vi "Game.vi"() -> ()   [LabVIEW 2025]
uses:
  Controls/Game.ctl
  Controls/Player.ctl
  <vilib>/Utility/miscctls.llb/LVPositionTypeDef.ctl
  38faf71d-537f-4ad3-ba2d-5a527e0ddfb2.vi
panel:
  out "CurrentPlayer":i32
  out "Hand3":u16[](array[ring]) caption="Tiles"
  out "River4":u16[][](array[ring]) caption="Tiles"
  out "Door4":u16[](array[ring]) caption="Tiles"
  out "Hand4":u16[](array[ring]) caption="Tiles"
  out "Door3":u16[](array[ring]) caption="Tiles"
  out "River 3":u16[][](array[ring]) caption="Tiles"
  in  "Chi 3":bool
  in  "Chi 2":bool
  in  "Chi 1":bool
  in  "Cancel":bool
  in  "Hu":bool
  in  "Kung":bool
  in  "Pong":bool
  in  "Chi":bool
  out "Players":T1[](array[typedef])
  out "Game":T2
  out "River1":u16[][](array[ring]) caption="Tiles"
  in  "Buttons":bool[](array[boolean])=[FALSE, FALSE, FALSE, FALSE, FALSE, FALSE, FALSE, FALSE, FALSE, FALSE, FALSE, FALSE, FALSE, FALSE, FALSE, FALSE, FALSE]
  out "Hand1":u16[](array[ring])
  out "River2":u16[][](array[ring]) caption="Tiles"
  out "Door2":u16[](array[ring]) caption="Tiles"
  out "Hand2":u16[](array[ring]) caption="Tiles"
  out "Door1":u16[](array[ring]) caption="Tiles"
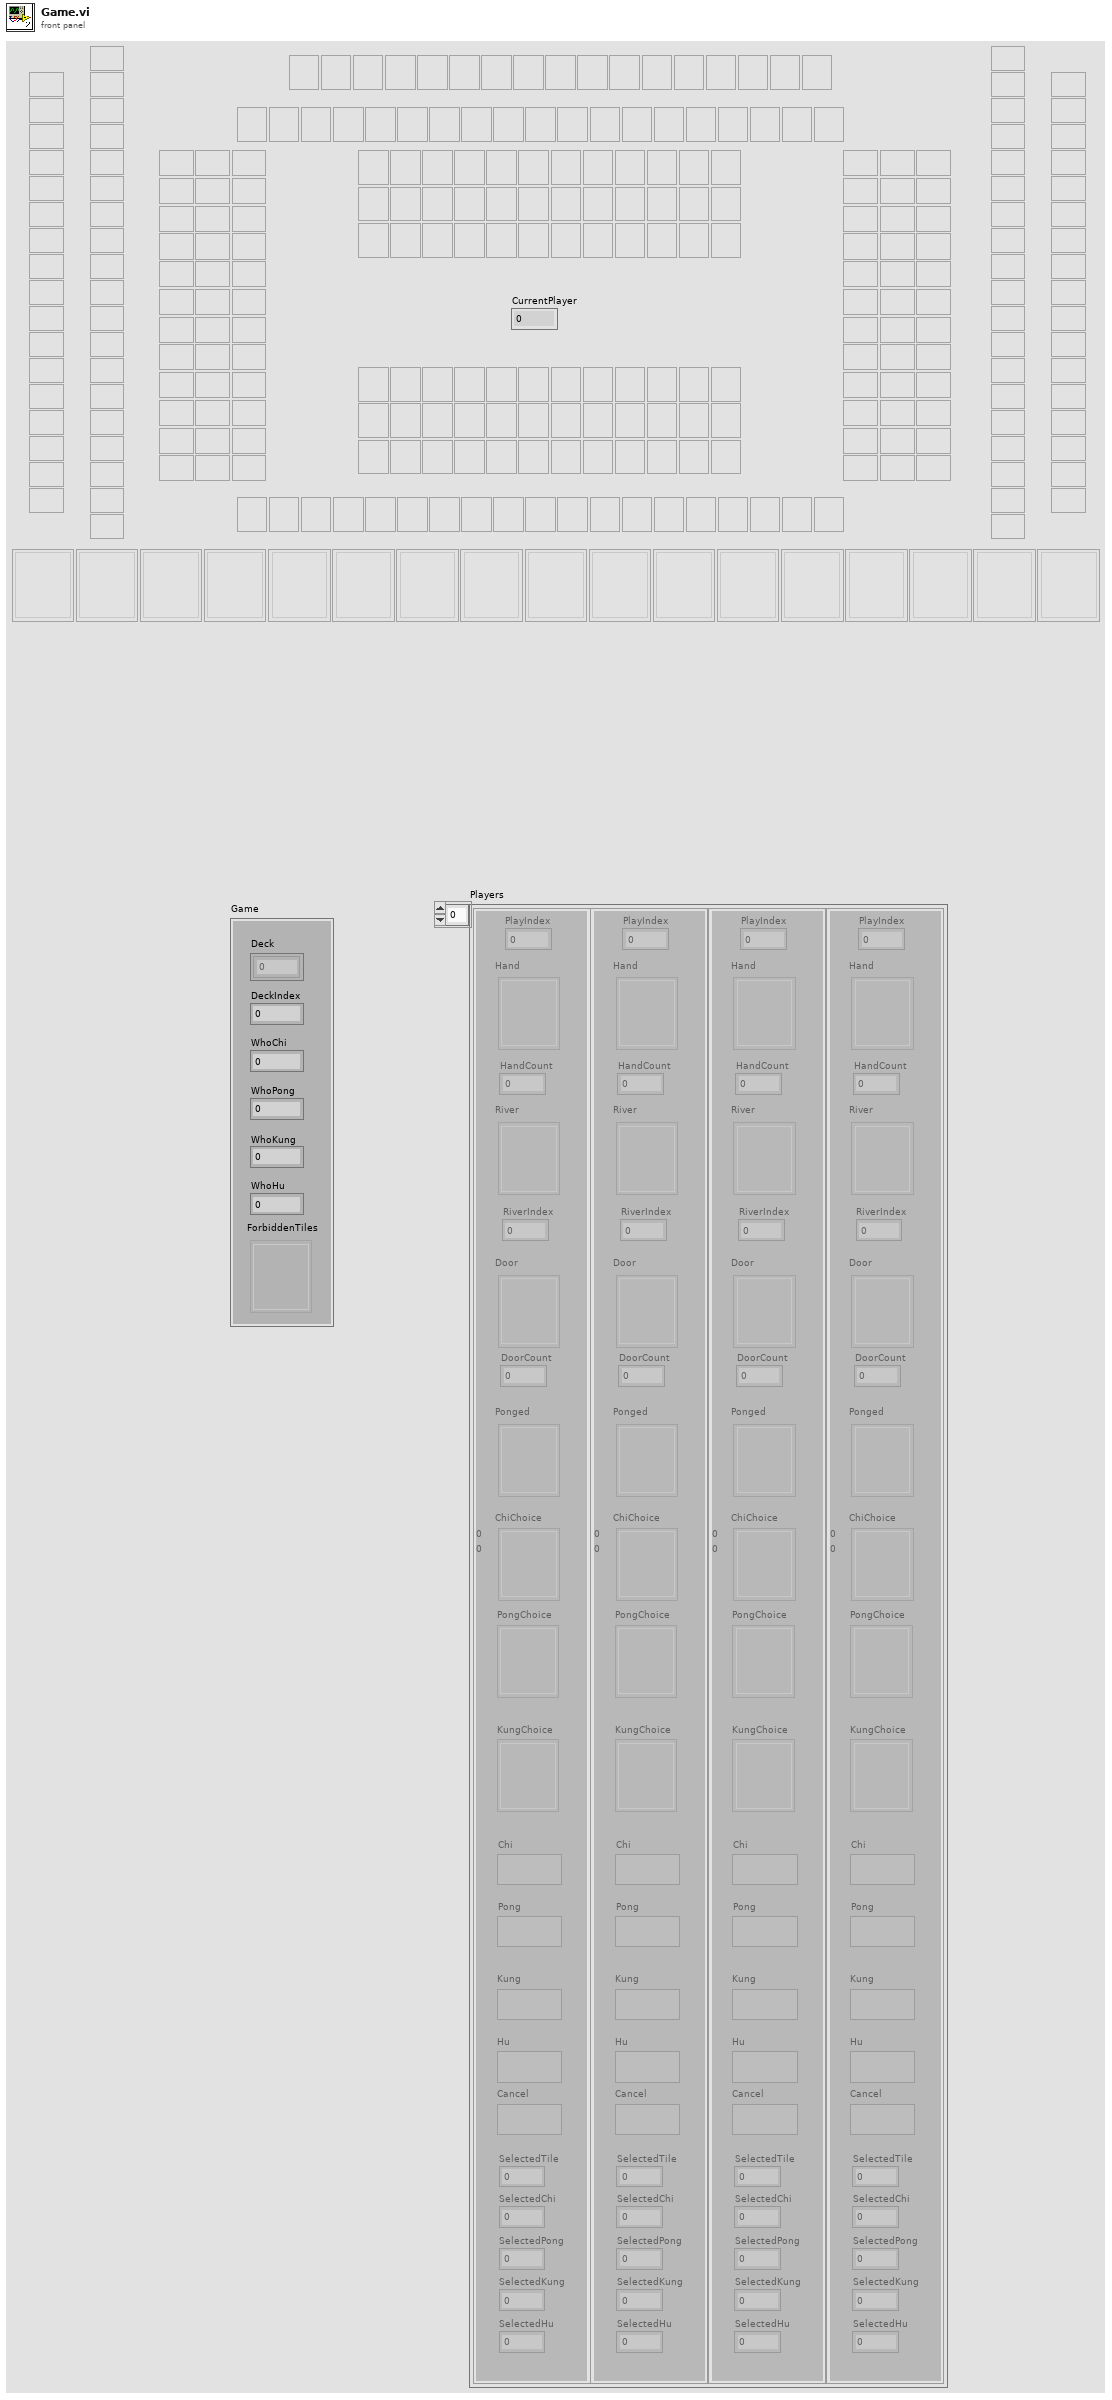
[diagram p1: front panel]
types:
  T1 = typedef "Player.ctl" = cluster{"PlayIndex":u16, "Hand":u16[], "HandCount":u16, "RiverIndex":u16, "Door":u16[], "DoorCount":u16, "Ponged":u16[], "ChiChoice":u16[][], "River":u16[][], "Chi":bool, "Pong":bool, "Kung":bool, "Hu":bool, "Cancel":bool, "PongChoice":u16, "KungChoice":u16, "SelectedTile":i16, "SelectedChi":i16, "SelectedPong":i16, "SelectedKung":i16, "SelectedHu":i16}
  T2 = typedef "Game.ctl" = cluster{"DeckIndex":u16, "Deck":u16[], "WhoChi":u16, "WhoPong":u16, "WhoKung":u16, "WhoHu":u16, "ForbiddenTiles":u16[]}
  T3 = enum16{"Game Start", "DeckSetup", "PlayerSetup", "Deal", "Game End", "Draw", "Wait", "WaitKung", "Throw", "Chi", "Pong", "Kung", "Hu", "Interrupt0", "Interrupt1", "Interrupt2", "Interrupt3", "Chi?", "Pong?", "Kung?", "Hu?"}
  T4 = enum8{"Enabled", "Disabled", "Disabled and Grayed Out"}
  T5 = typedef "LVPositionTypeDef.ctl" = cluster{"Left":i32, "Top":i32}
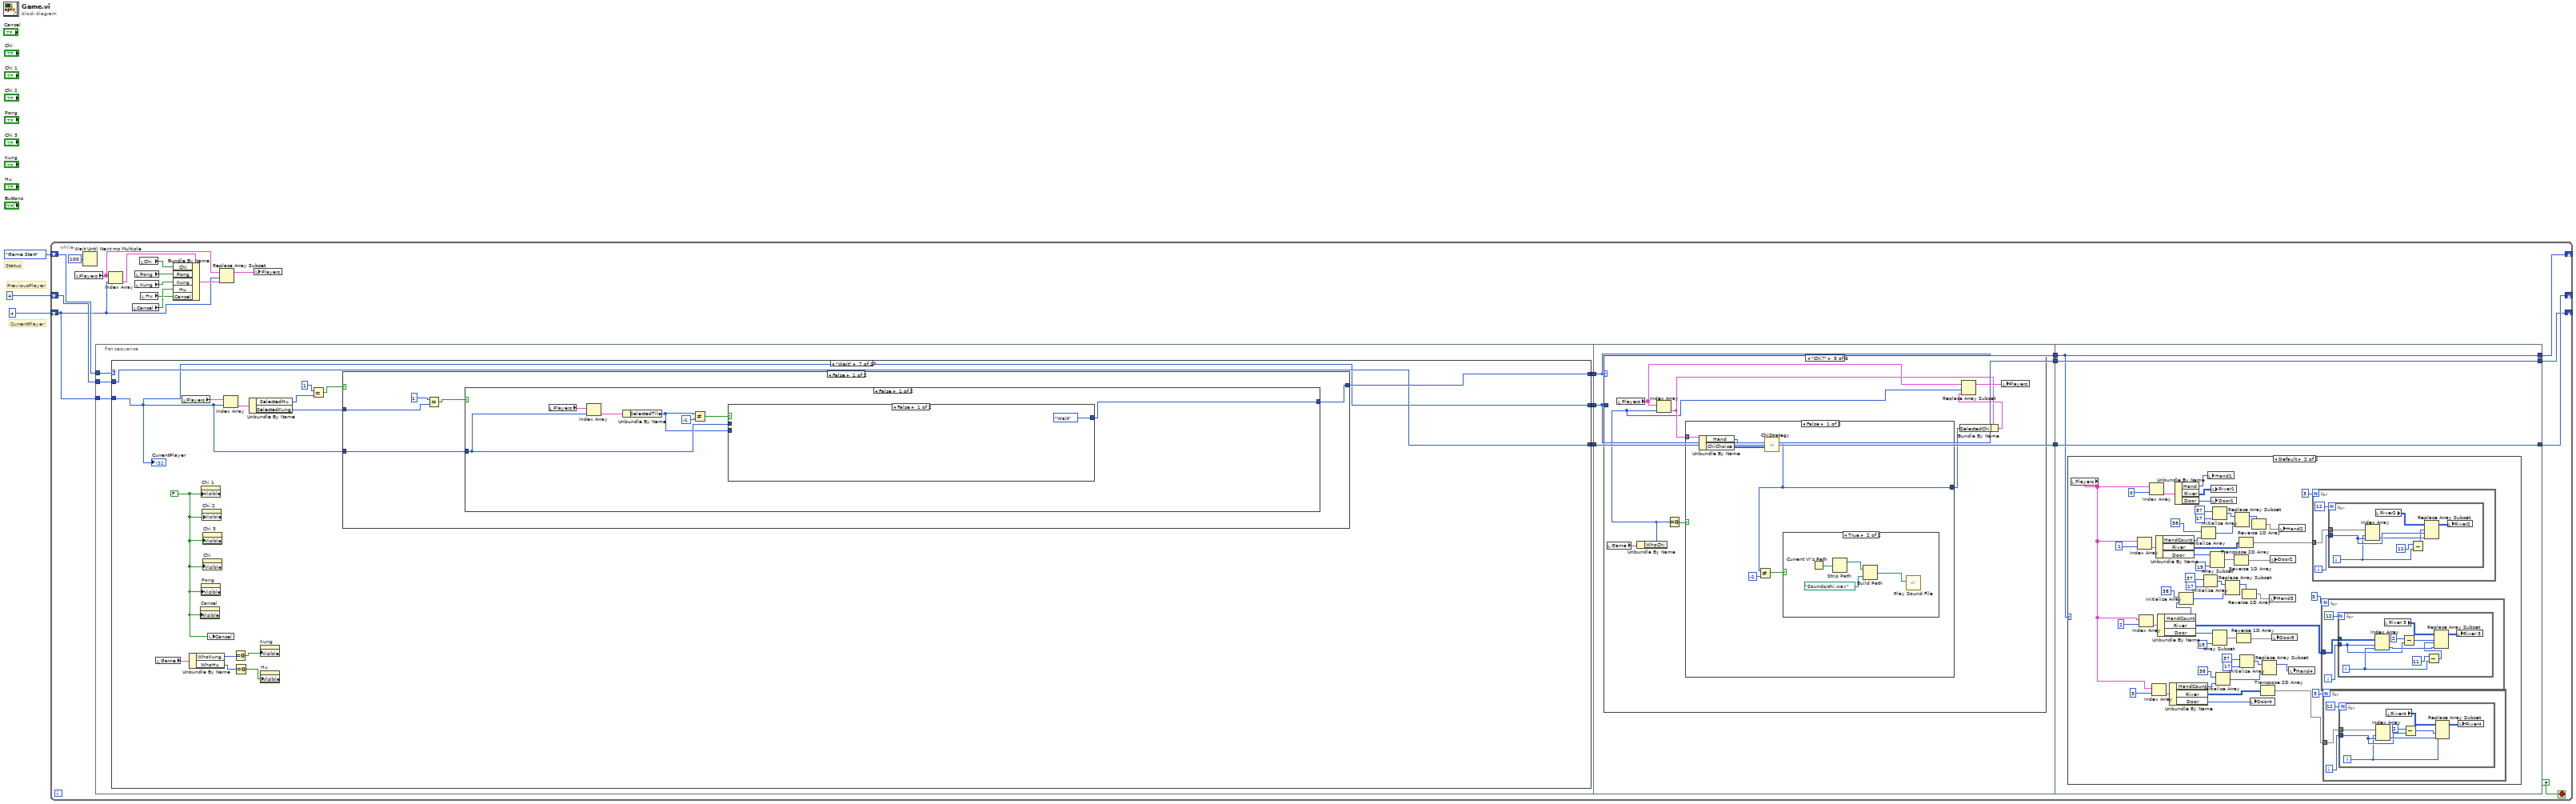
[diagram p0: block diagram]
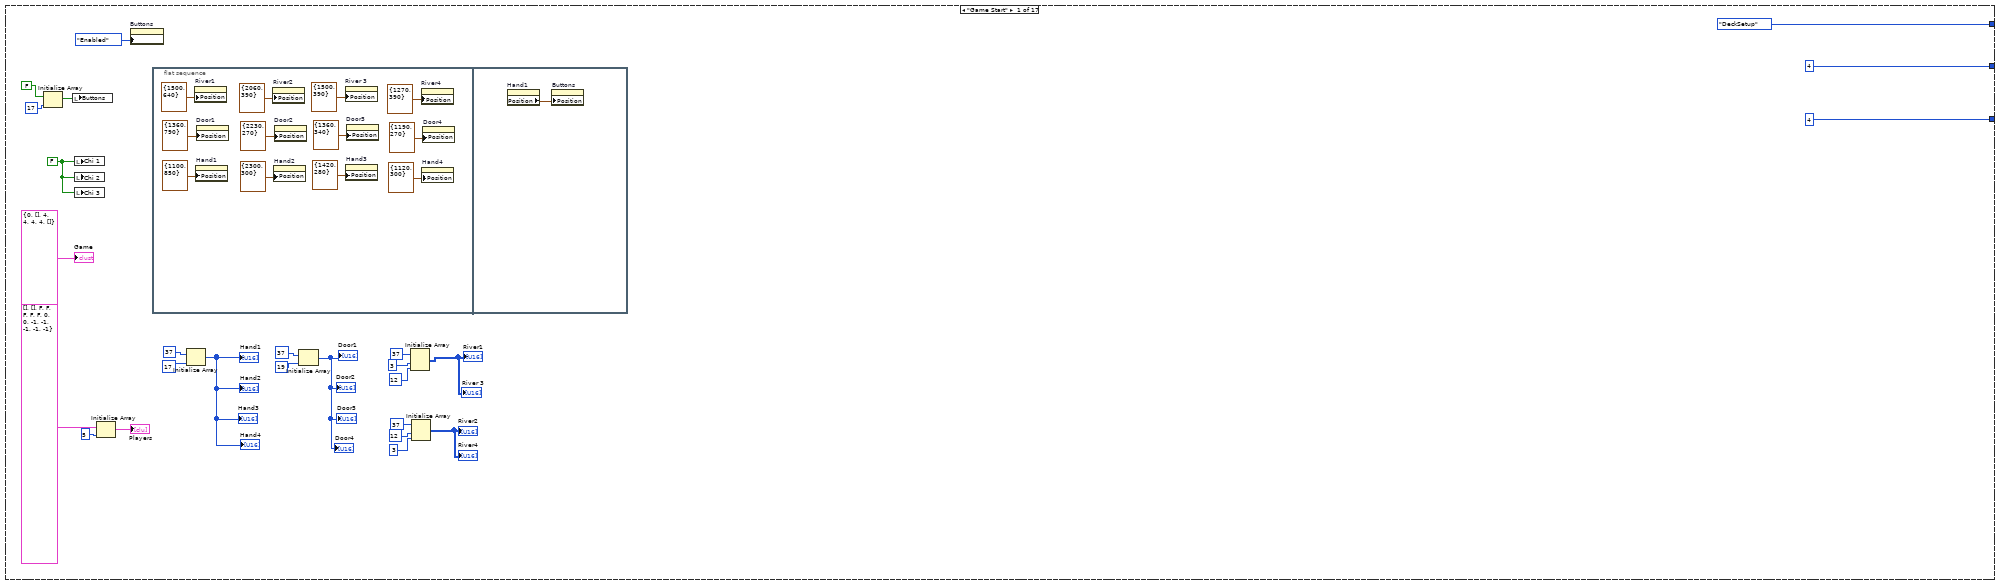
[diagram p2: hidden frame]
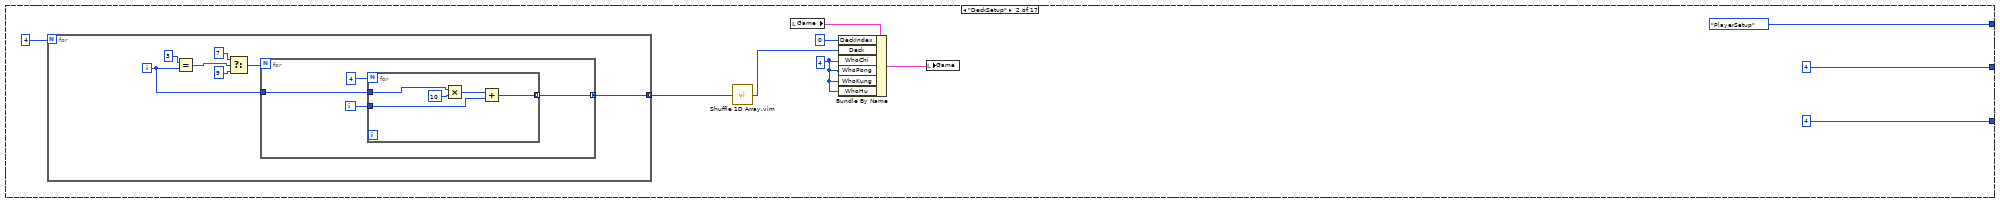
[diagram p3: hidden frame]
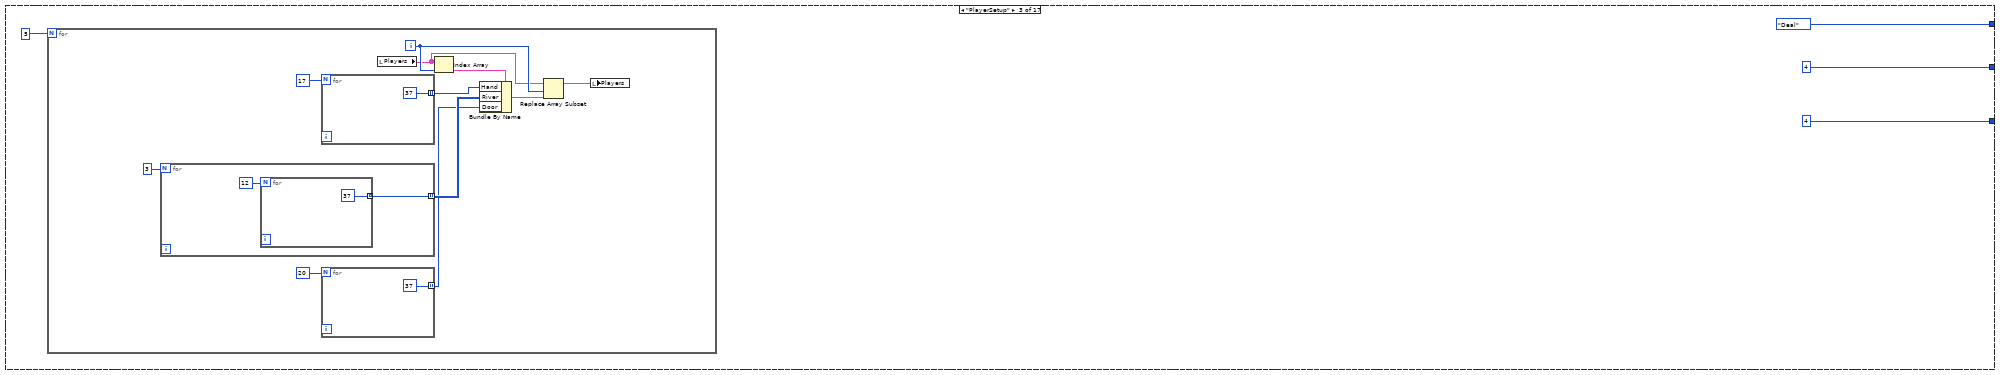
[diagram p4: hidden frame]
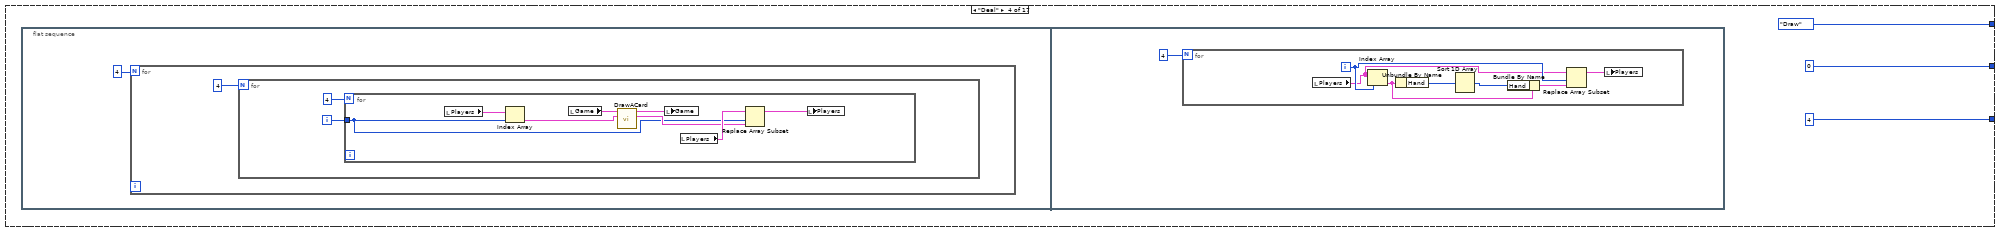
[diagram p5: hidden frame]
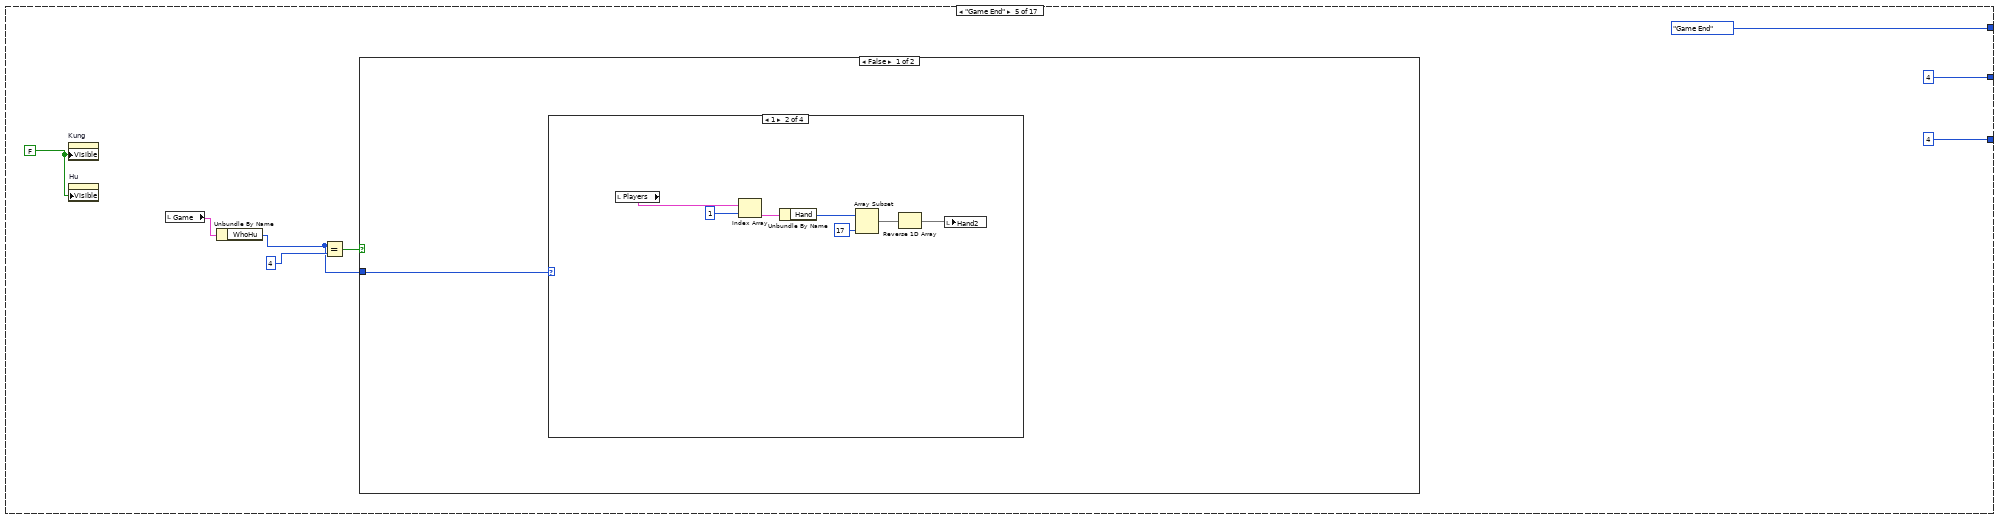
[diagram p6: hidden frame]
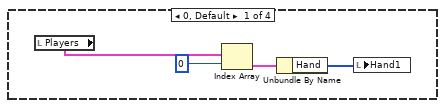
[diagram p7: hidden frame]
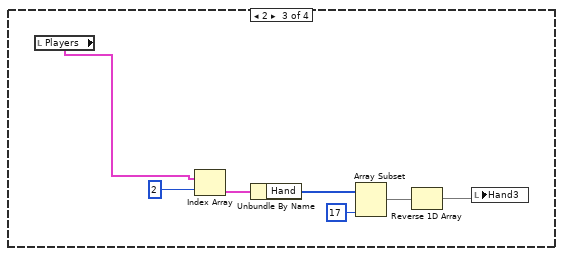
[diagram p8: hidden frame]
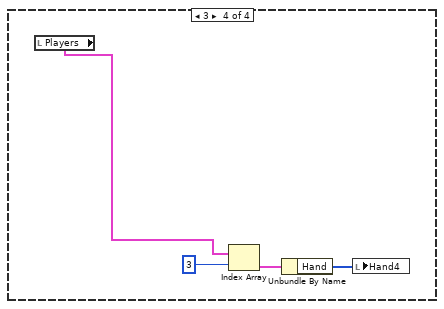
[diagram p9: hidden frame]
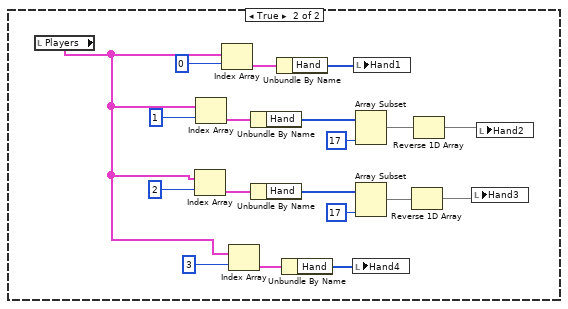
[diagram p10: hidden frame]
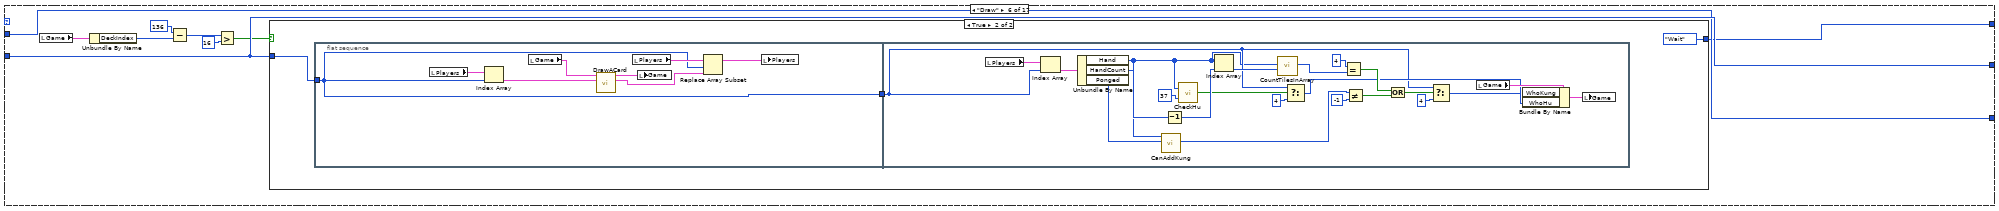
[diagram p11: hidden frame]
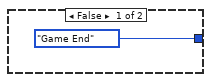
[diagram p12: hidden frame]
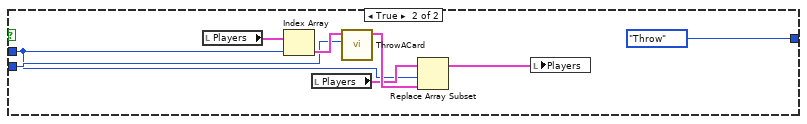
[diagram p13: hidden frame]
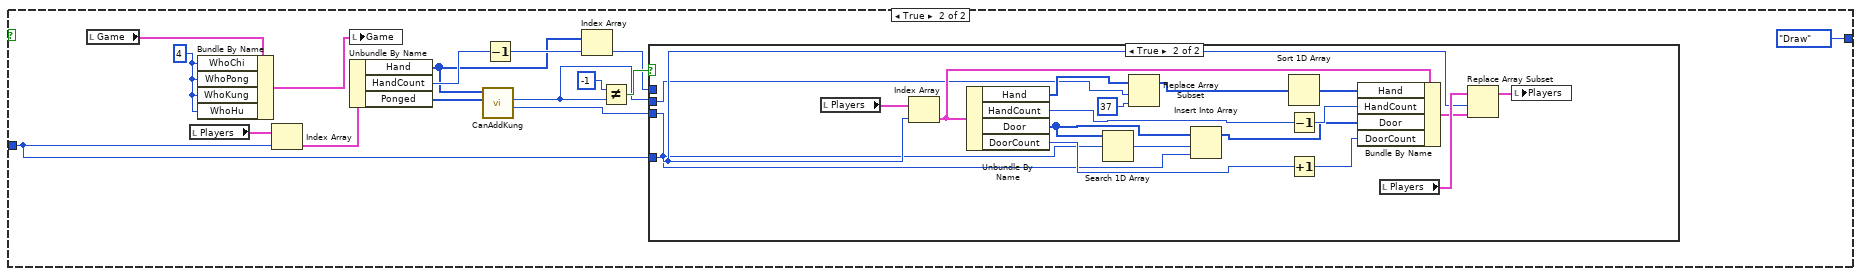
[diagram p14: hidden frame]
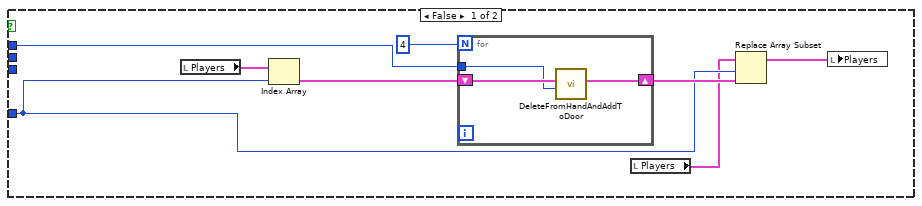
[diagram p15: hidden frame]
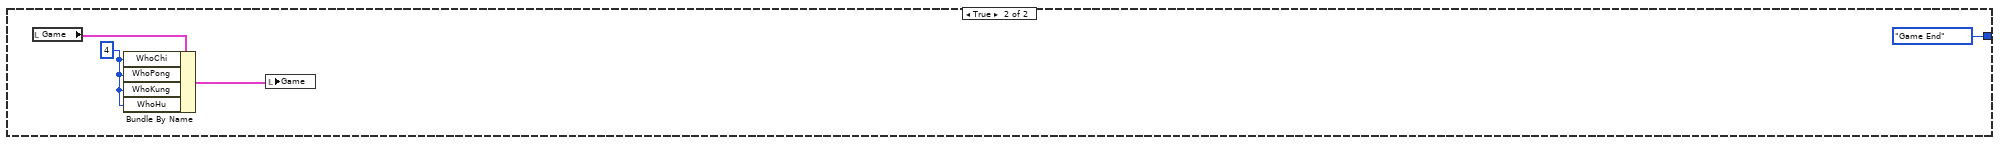
[diagram p16: hidden frame]
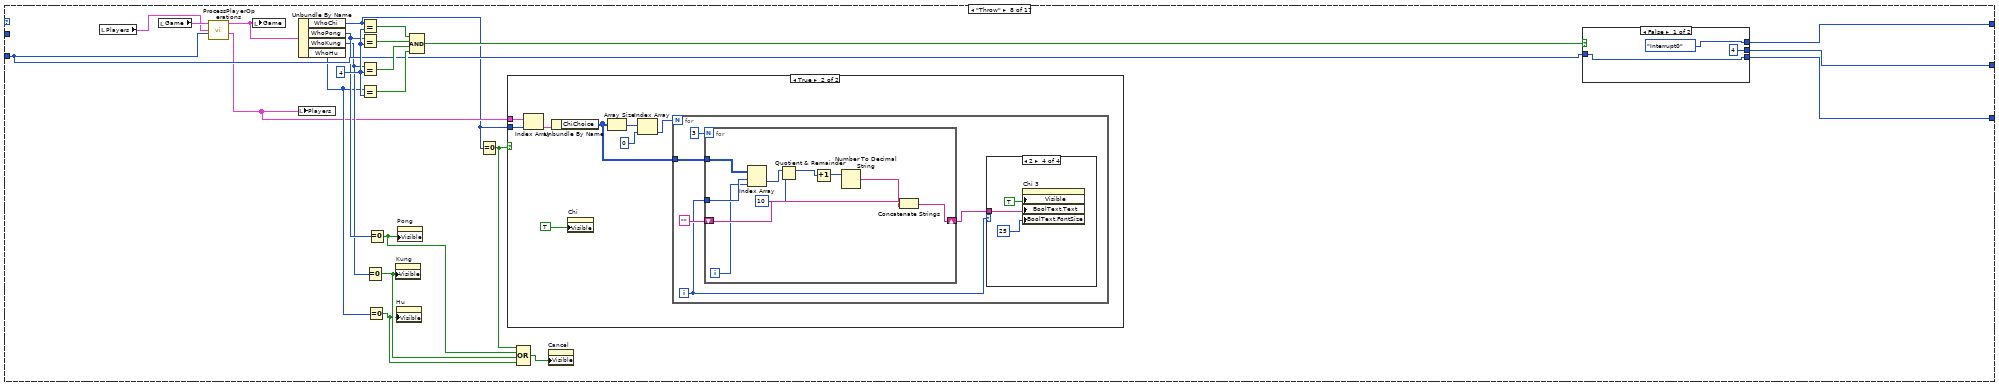
[diagram p17: hidden frame]
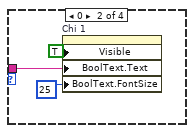
[diagram p20: hidden frame]
diagram:
  # "PreviousPlayer"
  # "CurrentPlayer"
  # "Status"
  n1 = while {
    shift-right: [w21] -> _
    shift-left: T3."Game Start" -> [w11]
    shift-right: [w22] -> _
    shift-left: 4 -> [w10]
    shift-right: [w23] -> _
    shift-left: 4 -> [w24]
    stop <- FALSE stop-if-true
    n2 = local read "Players"() -> (w18:T1[])
    n3 = Wait Until Next ms Multiple(millisecond multiple=100) -> ()  [unwired: 1 out]
    n4 = flat-sequence {
      tunnel: w24 -> [w32]
      tunnel: w11 -> [w29]
      tunnel: w10 -> [w28]
      tunnel: [w31] -> w9
      tunnel: [w27] -> w8
      tunnel: [w30] -> w7
      tunnel: w9 -> [w573]
      tunnel: w8 -> [w572]
      tunnel: w7 -> [w574]
      tunnel: [w573] -> w6
      tunnel: [w572] -> w5
      tunnel: [w574] -> w4
      tunnel: [w779] -> w21
      tunnel: [w780] -> w22
      tunnel: [w781] -> w23
      tunnel: w6 -> [w781]
      tunnel: w5 -> [w780]
      tunnel: w4 -> [w779]
      frame #0 {
        n5 = case shown="\"Wait\"" w29 {
          tunnel: [T3."DeckSetup" T3."PlayerSetup" T3."Deal" T3."Draw" T3."Game End" w191 w249 w336 w385 w396 w407 w419 w433 w484 w522 w556 T3."Game End"] -> w30
          tunnel: w28 -> [_ _ _ _ _ w199 w246 w334 _ _ _ _ w431 w480 w518 w552 _]
          tunnel: w32 -> [_ _ _ _ _ w198 w248 _ w386 w395 w409 w418 w434 w481 w519 w553 _]
          tunnel: [4 4 4 4 4 w198 w248 w335 w386 w395 w409 w420 w432 w483 w521 w555 4] -> w31
          tunnel: [4 4 4 0 4 w199 w246 w337 w384 w397 w406 w417 w436 w482 w520 w554 4] -> w27
          frame "Game Start" {
            w51 = FALSE
            n6 = Initialize Array(FALSE, 17) -> (w48:bool[])
            n7 = local write "Buttons"(w48) -> ()
            n8 = local write "Chi 1"(w51) -> ()
            n9 = local write "Chi 2"(w51) -> ()
            n10 = local write "Chi 3"(w51) -> ()
            n11 = Initialize Array(T1 {"PlayIndex"=0, "Hand"=[], "HandCount"=0, "RiverIndex"=0, "Door"=[], "DoorCount"=0, "Ponged"=[], "ChiChoice"=[], "River"=[], "Chi"=FALSE, "Pong"=FALSE, "Kung"=FALSE, "Hu"=FALSE, "Cancel"=FALSE, "PongChoice"=0, "KungChoice"=0, "SelectedTile"=-1, "SelectedChi"=-1, "SelectedPong"=-1, "SelectedKung"=-1, "SelectedHu"=-1} ("element"), 5) -> (→"Players":T1[])
            n12 = property on="Buttons" class="Arr (strict)"("DisabledEnum"=T4."Enabled" ("Disabled")) -> ()  [unwired: 2 in, 2 out]
            n13 = flat-sequence {
              frame #0 {
                n14 = property on="River1" class="Arr (strict)"("Position"=T5 {"Left"=1500, "Top"=640}) -> ()  [unwired: 2 in, 2 out]
                n15 = property on="Hand1" class="Arr (strict)"("Position"=T5 {"Left"=1100, "Top"=850}) -> ()  [unwired: 2 in, 2 out]
                n16 = property on="Door1" class="Arr (strict)"("Position"=T5 {"Left"=1360, "Top"=790}) -> ()  [unwired: 2 in, 2 out]
                n17 = property on="River2" class="Arr (strict)"("Position"=T5 {"Left"=2060, "Top"=390}) -> ()  [unwired: 2 in, 2 out]
                n18 = property on="Hand2" class="Arr (strict)"("Position"=T5 {"Left"=2300, "Top"=300}) -> ()  [unwired: 2 in, 2 out]
                n19 = property on="Door2" class="Arr (strict)"("Position"=T5 {"Left"=2230, "Top"=270}) -> ()  [unwired: 2 in, 2 out]
                n20 = property on="River 3" class="Arr (strict)"("Position"=T5 {"Left"=1500, "Top"=390}) -> ()  [unwired: 2 in, 2 out]
                n21 = property on="Hand3" class="Arr (strict)"("Position"=T5 {"Left"=1420, "Top"=280}) -> ()  [unwired: 2 in, 2 out]
                n22 = property on="Door3" class="Arr (strict)"("Position"=T5 {"Left"=1360, "Top"=340}) -> ()  [unwired: 2 in, 2 out]
                n23 = property on="River4" class="Arr (strict)"("Position"=T5 {"Left"=1270, "Top"=390}) -> ()  [unwired: 2 in, 2 out]
                n24 = property on="Hand4" class="Arr (strict)"("Position"=T5 {"Left"=1120, "Top"=300}) -> ()  [unwired: 2 in, 2 out]
                n25 = property on="Door4" class="Arr (strict)"("Position"=T5 {"Left"=1190, "Top"=270}) -> ()  [unwired: 2 in, 2 out]
              }
              frame #1 {
                n26 = property on="Hand1" class="Arr (strict)"() -> ("Position"=w71:T5)  [unwired: 2 in, 2 out]
                n27 = property on="Buttons" class="Arr (strict)"("Position"=w71) -> ()  [unwired: 2 in, 2 out]
              }
            }
            n28 = Initialize Array(37, 17) -> (→"Hand1" →"Hand3" →"Hand4" →"Hand2":i32[])
            n29 = Initialize Array(37, 19) -> (→"Door3" →"Door1" →"Door4" →"Door2":i32[])
            n30 = Initialize Array(37, 3, 12) -> (→"River1" →"River 3":i32[][])
            n31 = Initialize Array(37, 12, 3) -> (→"River2" →"River4":i32[][])
            "Game" <- T2 {"DeckIndex"=0, "Deck"=[], "WhoChi"=4, "WhoPong"=4, "WhoKung"=4, "WhoHu"=4, "ForbiddenTiles"=[]} ("Game")
          }
          frame "DeckSetup" {
            w72 = 4
            n32 = for {
              N: 4 -> [_]
              tunnel: [w85] -> w81 mode=concatenating
              i -> [w83]
              n33 = Equal?(x=3, y=w83) -> (x = y?=w84:bool)
              n34 = Select(t=7, s=w84, f=9) -> (s? t:f=w87:i32)
              n35 = for {
                N: w87 -> [_]
                tunnel: w83 -> [w92]
                tunnel: [w90] -> w85 mode=concatenating
                i -> [w91]
                n36 = for {
                  N: 4 -> [_]
                  tunnel: w92 -> [w95]
                  tunnel: w91 -> [w94]
                  tunnel: [w93] -> w90 mode=indexing
                  n37 = Multiply(x=w95, y=10) -> (x*y=w97:i32)
                  n38 = Add(x=w97, y=w94) -> (x+y=w93:i32)
                }
              }
            }
            n39 = call "Shuffle 1D Array.vim"("array"=w81) -> ("shuffled array"=w78:i32[])  [unwired: 4 in]
            n40 = local read "Game"() -> (w79:T2)
            n41 = Bundle By Name(cluster=w79, "DeckIndex"=0, "Deck"=w78, "WhoChi"=w72, "WhoPong"=w72, "WhoKung"=w72, "WhoHu"=w72) -> (w80:T2)
            n42 = local write "Game"(w80) -> ()
          }
          frame "PlayerSetup" {
            n43 = for {
              N: 5 -> [_]
              i -> [w109]
              n44 = for {
                N: 3 -> [_]
                tunnel: [w115] -> w105 mode=indexing
                n45 = for {
                  N: 12 -> [_]
                  tunnel: [37] -> w115 mode=indexing
                }
              }
              n46 = for {
                N: 17 -> [_]
                tunnel: [37] -> w106 mode=indexing
              }
              n47 = for {
                N: 20 -> [_]
                tunnel: [37] -> w102 mode=indexing
              }
              n48 = local read "Players"() -> (w108:T1[])
              n49 = Index Array(array=w108, index=w109) -> (element=w112:T1)
              n50 = Bundle By Name(cluster=w112, "Hand"=w106, "River"=w105, "Door"=w102) -> (w111:T1)
              n51 = Replace Array Subset(array=w108, new element=w111, index=w109) -> (w110:T1[])
              n52 = local write "Players"(w110) -> ()
            }
          }
          frame "Deal" {
            n53 = flat-sequence {
              frame #0 {
                n54 = for {
                  N: 4 -> [_]
                  n55 = for {
                    N: 4 -> [_]
                    i -> [w123]
                    n56 = for {
                      N: 4 -> [_]
                      tunnel: w123 -> [w127]
                      n57 = local read "Players"() -> (w126:T1[])
                      n58 = Index Array(array=w126, index=w127) -> (element=w125:T1)
                      n59 = local read "Game"() -> (w128:T2)
                      n60 = call "DrawACard.vi"("Player"=w125, "Game"=w128) -> ("NewPlayer"=w130:T1, "NewGame"=w132:T2)  [unwired: 8 in]
                      n61 = local write "Game"(w132) -> ()
                      n62 = local read "Players"() -> (w131:T1[])
                      n63 = Replace Array Subset(array=w131, new element=w130, index=w127) -> (w129:T1[])
                      n64 = local write "Players"(w129) -> ()
                    }
                  }
                }
              }
              frame #1 {
                n65 = for {
                  N: 4 -> [_]
                  i -> [w135]
                  n66 = local read "Players"() -> (w134:T1[])
                  n67 = Index Array(array=w134, index=w135) -> (element=w140:T1)
                  n68 = Unbundle By Name(w140) -> ("Hand"=w139:u16[])
                  n69 = Sort 1D Array(array=w139) -> (sorted array=w138:u16[])
                  n70 = Bundle By Name(cluster=w140, "Hand"=w138) -> (w136:T1)
                  n71 = Replace Array Subset(array=w134, new element=w136, index=w135) -> (w137:T1[])
                  n72 = local write "Players"(w137) -> ()
                }
              }
            }
          }
          frame "Game End" {
            w141 = FALSE
            n73 = property on="Kung" class="Bool (strict)"("Visible"=w141) -> ()  [unwired: 2 in, 2 out]
            n74 = property on="Hu" class="Bool (strict)"("Visible"=w141) -> ()  [unwired: 2 in, 2 out]
            n75 = local read "Game"() -> (w145:T2)
            n76 = Unbundle By Name(w145) -> ("WhoHu"=w142:u16)
            n77 = Equal?(x=w142, y=4) -> (x = y?=w144:bool)
            n78 = case shown="False" w144 {
              tunnel: w142 -> [w149 _]
              frame False {
                n79 = case shown="1" w149 {
                  frame 0, Default {
                    n80 = local read "Players"() -> (w153:T1[])
                    n81 = Index Array(array=w153, index=0) -> (element=w151:T1)
                    n82 = Unbundle By Name(w151) -> ("Hand"=w152:u16[])
                    n83 = local write "Hand1"(w152) -> ()
                  }
                  frame 1 {
                    n84 = local read "Players"() -> (w156:T1[])
                    n85 = Index Array(array=w156, index=1) -> (element=w155:T1)
                    n86 = Unbundle By Name(w155) -> ("Hand"=w154:u16[])
                    n87 = Array Subset(array=w154, length=17) -> (w157:u16[])  [unwired: 1 in]
                    n88 = Reverse 1D Array(array=w157) -> (reversed array=w158:u16[])
                    n89 = local write "Hand2"(w158) -> ()
                  }
                  frame 2 {
                    n90 = local read "Players"() -> (w161:T1[])
                    n91 = Index Array(array=w161, index=2) -> (element=w162:T1)
                    n92 = Unbundle By Name(w162) -> ("Hand"=w163:u16[])
                    n93 = Array Subset(array=w163, length=17) -> (w164:u16[])  [unwired: 1 in]
                    n94 = Reverse 1D Array(array=w164) -> (reversed array=w165:u16[])
                    n95 = local write "Hand3"(w165) -> ()
                  }
                  frame 3 {
                    n96 = local read "Players"() -> (w170:T1[])
                    n97 = Index Array(array=w170, index=3) -> (element=w169:T1)
                    n98 = Unbundle By Name(w169) -> ("Hand"=w168:u16[])
                    n99 = local write "Hand4"(w168) -> ()
                  }
                }
              }
              frame True {
                n100 = local read "Players"() -> (w182:T1[])
                n101 = Index Array(array=w182, index=2) -> (element=w188:T1)
                n102 = Index Array(array=w182, index=1) -> (element=w185:T1)
                n103 = Index Array(array=w182, index=0) -> (element=w190:T1)
                n104 = Index Array(array=w182, index=3) -> (element=w183:T1)
                n105 = Unbundle By Name(w185) -> ("Hand"=w186:u16[])
                n106 = Unbundle By Name(w188) -> ("Hand"=w187:u16[])
                n107 = Unbundle By Name(w190) -> ("Hand"=w189:u16[])
                n108 = Unbundle By Name(w183) -> ("Hand"=w184:u16[])
                n109 = local write "Hand4"(w184) -> ()
                n110 = local write "Hand1"(w189) -> ()
                n111 = Array Subset(array=w186, length=17) -> (w175:u16[])  [unwired: 1 in]
                n112 = Array Subset(array=w187, length=17) -> (w174:u16[])  [unwired: 1 in]
                n113 = Reverse 1D Array(array=w174) -> (reversed array=w172:u16[])
                n114 = Reverse 1D Array(array=w175) -> (reversed array=w173:u16[])
                n115 = local write "Hand3"(w172) -> ()
                n116 = local write "Hand2"(w173) -> ()
              }
            }
          }
          frame "Draw" {
            n117 = local read "Game"() -> (w196:T2)
            n118 = Unbundle By Name(w196) -> ("DeckIndex"=w195:u16)
            n119 = Subtract(x=136, y=w195) -> (x-y=w194:i32)
            n120 = Greater?(x=w194, y=16) -> (0:w193:bool)
            n121 = case shown="True" w193 {
              tunnel: w199 -> [_ w203]
              tunnel: [T3."Game End" T3."Wait"] -> w191
              frame False {
              }
              frame True {
                n122 = flat-sequence {
                  tunnel: w203 -> [w204]
                  tunnel: [w204] -> w201
                  tunnel: w201 -> [w217]
                  frame #0 {
                    n123 = local read "Players"() -> (w211:T1[])
                    n124 = Index Array(array=w211, index=w204) -> (element=w210:T1)
                    n125 = local read "Game"() -> (w209:T2)
                    n126 = call "DrawACard.vi"("Player"=w210, "Game"=w209) -> ("NewPlayer"=w206:T1, "NewGame"=w207:T2)  [unwired: 8 in]
                    n127 = local read "Players"() -> (w208:T1[])
                    n128 = local write "Game"(w207) -> ()
                    n129 = Replace Array Subset(array=w208, new element=w206, index=w204) -> (w205:T1[])
                    n130 = local write "Players"(w205) -> ()
                  }
                  frame #1 {
                    n131 = local read "Players"() -> (w218:T1[])
                    n132 = Index Array(array=w218, index=w217) -> (element=w234:T1)
                    n133 = Unbundle By Name(w234) -> ("Hand"=w212:u16[], "HandCount"=w233:u16, "Ponged"=w216:u16[])
                    n134 = call "CanAddKung.vi"("Ponged"=w216, "Hand"=w212) -> ("HandIndex"=w215:i16)  [unwired: 8 in, 1 out]
                    n135 = Decrement(x=w233) -> (x-1=w232:u16)
                    n136 = call "CheckHu.vi"("TargetTile"=37, "Hand"=w212) -> ("CanHu"=w222:bool)
                    n137 = Index Array(array=w212, index=w232) -> (element=w229:u16)
                    n138 = call "CountTilesInArray.vi"("Tile"=w229, "Hand"=w212) -> ("Count"=w230:u16)  [unwired: 9 in]
                    n139 = Select(t=w217, s=w222, f=4) -> (s? t:f=w220:i32)
                    n140 = Equal?(x=4, y=w230) -> (x = y?=w231:bool)
                    n141 = Not Equal?(x=w215, y=-1) -> (x != y?=w213:bool)
                    n142 = Or(x=w231, y=w213) -> (x .or. y?=w225:bool)
                    n143 = Select(t=w217, s=w225, f=4) -> (s? t:f=w219:i32)
                    n144 = local read "Game"() -> (w227:T2)
                    n145 = Bundle By Name(cluster=w227, "WhoKung"=w219, "WhoHu"=w220) -> (w226:T2)
                    n146 = local write "Game"(w226) -> ()
                  }
                }
              }
            }
          }
          frame "Wait" {
            w235 = FALSE
            n147 = local read "Game"() -> (w240:T2)
            n148 = local read "Players"() -> (w247:T1[])
            n149 = Unbundle By Name(w240) -> ("WhoKung"=w239:u16, "WhoHu"=w237:u16)
            n150 = property on="Cancel" class="Bool (strict)"("Visible"=w235) -> ()  [unwired: 2 in, 2 out]
            n151 = property on="Chi 1" class="Bool (strict)"("Visible"=w235) -> ()  [unwired: 2 in, 2 out]
            n152 = property on="Pong" class="Bool (strict)"("Visible"=w235) -> ()  [unwired: 2 in, 2 out]
            n153 = property on="Chi 2" class="Bool (strict)"("Visible"=w235) -> ()  [unwired: 2 in, 2 out]
            n154 = property on="Chi 3" class="Bool (strict)"("Visible"=w235) -> ()  [unwired: 2 in, 2 out]
            n155 = property on="Chi" class="Bool (strict)"("Visible"=w235) -> ()  [unwired: 2 in, 2 out]
            n156 = local write "Cancel"(w235) -> ()
            n157 = Index Array(array=w247, index=w246) -> (element=w245:T1)
            n158 = Equal To 0?(x=w239) -> (x = 0?=w238:bool)
            n159 = Equal To 0?(x=w237) -> (x = 0?=w236:bool)
            n160 = Unbundle By Name(w245) -> ("SelectedHu"=w243:i16, "SelectedKung"=w244:i16)
            n161 = property on="Kung" class="Bool (strict)"("Visible"=w238) -> ()  [unwired: 2 in, 2 out]
            n162 = property on="Hu" class="Bool (strict)"("Visible"=w236) -> ()  [unwired: 2 in, 2 out]
            n163 = Equal?(x=1, y=w243) -> (x = y?=w242:bool)
            n164 = case shown="False" w242 {
              tunnel: [w254 T3."Game End"] -> w249
              tunnel: w246 -> [w253 _]
              tunnel: w244 -> [w252 _]
              frame False {
                n165 = Equal?(x=1, y=w252) -> (x = y?=w250:bool)
                n166 = case shown="False" w250 {
                  tunnel: [w261 T3."Draw"] -> w254
                  tunnel: w253 -> [w259 w280]
                  frame False {
                    n167 = local read "Players"() -> (w260:T1[])
                    n168 = Index Array(array=w260, index=w259) -> (element=w258:T1)
                    n169 = Unbundle By Name(w258) -> ("SelectedTile"=w257:i16)
                    n170 = Not Equal?(x=w257, y=-1) -> (x != y?=w255:bool)
                    n171 = case shown="False" w255 {
                      tunnel: [T3."Wait" T3."Throw"] -> w261
                      tunnel: w259 -> [_ w264]
                      tunnel: w257 -> [_ w268]
                      frame False {
                      }
                      frame True {
                        n172 = local read "Players"() -> (w270:T1[])
                        n173 = Index Array(array=w270, index=w264) -> (element=w269:T1)
                        n174 = local read "Players"() -> (w266:T1[])
                        n175 = call "ThrowACard.vi"("SelectedIndex"=w268, "Player"=w269) -> ("NewPlayer"=w267:T1)  [unwired: 9 in]
                        n176 = Replace Array Subset(array=w266, new element=w267, index=w264) -> (w265:T1[])
                        n177 = local write "Players"(w265) -> ()
                      }
                    }
                  }
                  frame True {
                    w275 = 4
                    n178 = local read "Game"() -> (w277:T2)
                    n179 = local read "Players"() -> (w281:T1[])
                    n180 = Bundle By Name(cluster=w277, "WhoChi"=w275, "WhoPong"=w275, "WhoKung"=w275, "WhoHu"=w275) -> (w276:T2)
                    n181 = Index Array(array=w281, index=w280) -> (element=w279:T1)
                    n182 = local write "Game"(w276) -> ()
                    n183 = Unbundle By Name(w279) -> ("Hand"=w272:u16[], "HandCount"=w278:u16, "Ponged"=w271:u16[])
                    n184 = call "CanAddKung.vi"("Ponged"=w271, "Hand"=w272) -> ("TIle"=w273:u16, "HandIndex"=w274:i16)  [unwired: 8 in]
                    n185 = Decrement(x=w278) -> (x-1=w285:u16)
                    n186 = Index Array(array=w272, index=w285) -> (element=w283:u16)
                    n187 = Not Equal?(x=-1, y=w274) -> (x != y?=w284:bool)
                    n188 = case shown="True" w284 {
                      tunnel: w280 -> [w289 w312]
                      tunnel: w283 -> [w291 _]
                      tunnel: w274 -> [_ w304]
                      tunnel: w273 -> [_ w298]
                      frame False {
                        n189 = local read "Players"() -> (w293:T1[])
                        n190 = Index Array(array=w293, index=w289) -> (element=w292:T1)
                        n191 = for {
                          N: 4 -> [_]
                          shift-right: [w295] -> w290
                          shift-left: w292 -> [w297]
                          tunnel: w291 -> [w296]
                          n192 = call "DeleteFromHandAndAddToDoor.vi"("Tile"=w296, "Player"=w297) -> ("NewPlayer"=w295:T1)  [unwired: 9 in]
                        }
                        n193 = local read "Players"() -> (w288:T1[])
                        n194 = Replace Array Subset(array=w288, new element=w290, index=w289) -> (w287:T1[])
                        n195 = local write "Players"(w287) -> ()
                      }
                      frame True {
                        n196 = local read "Players"() -> (w316:T1[])
                        n197 = Index Array(array=w316, index=w312) -> (element=w315:T1)
                        n198 = Unbundle By Name(w315) -> ("Hand"=w305:u16[], "HandCount"=w308:u16, "Door"=w302:u16[], "DoorCount"=w306:u16)
                        n199 = Search 1D Array(1D array=w302, element=w298) -> (index of element=w303:i32)  [unwired: 1 in]
                        n200 = Replace Array Subset(array=w305, new element=37, index=w304) -> (w300:u16[])
                        n201 = Insert Into Array(array=w302, index=w303, new element=w298) -> (w301:u16[])
                        n202 = Sort 1D Array(array=w300) -> (sorted array=w299:u16[])
                        n203 = Decrement(x=w308) -> (x-1=w309:u16)
                        n204 = Increment(x=w306) -> (x+1=w307:u16)
                        n205 = Bundle By Name(cluster=w315, "Hand"=w299, "HandCount"=w309, "Door"=w301, "DoorCount"=w307) -> (w313:T1)
                        n206 = local read "Players"() -> (w314:T1[])
                        n207 = Replace Array Subset(array=w314, new element=w313, index=w312) -> (w311:T1[])
                        n208 = local write "Players"(w311) -> ()
                      }
                    }
                  }
                }
              }
              frame True {
                w317 = 4
                n209 = local read "Game"() -> (w320:T2)
                n210 = Bundle By Name(cluster=w320, "WhoChi"=w317, "WhoPong"=w317, "WhoKung"=w317, "WhoHu"=w317) -> (w319:T2)
                n211 = local write "Game"(w319) -> ()
              }
            }
            "CurrentPlayer" <- w246
          }
          frame "Throw" {
            w339 = 4
            n212 = local read "Players"() -> (w331:T1[])
            n213 = local read "Game"() -> (w333:T2)
            n214 = call "ProcessPlayerOperations.vi"("WhoseTurn"=w334, "Players"=w331, "Game"=w333) -> ("NewPlayers"=w327:T1[], "NewGame"=w332:T2)  [unwired: 7 in]
            n215 = local write "Game"(w332) -> ()
            n216 = Unbundle By Name(w332) -> ("WhoChi"=w326:u16, "WhoPong"=w330:u16, "WhoKung"=w329:u16, "WhoHu"=w328:u16)
            n217 = local write "Players"(w327) -> ()
            n218 = Equal?(x=w326, y=w339) -> (x = y?=w343:bool)
            n219 = Equal?(x=w330, y=w339) -> (x = y?=w342:bool)
            n220 = Equal?(x=w329, y=w339) -> (x = y?=w341:bool)
            n221 = Equal?(x=w328, y=w339) -> (x = y?=w340:bool)
            n222 = Equal To 0?(x=w329) -> (x = 0?=w323:bool)
            n223 = Equal To 0?(x=w328) -> (x = 0?=w322:bool)
            n224 = Equal To 0?(x=w330) -> (x = 0?=w324:bool)
            n225 = property on="Kung" class="Bool (strict)"("Visible"=w323) -> ()  [unwired: 2 in, 2 out]
            n226 = property on="Hu" class="Bool (strict)"("Visible"=w322) -> ()  [unwired: 2 in, 2 out]
            n227 = property on="Pong" class="Bool (strict)"("Visible"=w324) -> ()  [unwired: 2 in, 2 out]
            n228 = Compound Arithmetic op=AND(w343, w342, w341, w340) -> (w338:bool)
            n229 = Equal To 0?(x=w326) -> (x = 0?=w325:bool)
            n230 = case shown="True" w325 {
              tunnel: w327 -> [_ w351]
              tunnel: w326 -> [_ w350]
              frame False {
              }
              frame True {
                n231 = Index Array(array=w351, index=w350) -> (element=w349:T1)
                n232 = Unbundle By Name(w349) -> ("ChiChoice"=w345:u16[][])
                n233 = property on="Chi" class="Bool (strict)"("Visible"=TRUE) -> ()  [unwired: 2 in, 2 out]
                n234 = Array Size(array=w345) -> (size(s)=w348:i32[])
                n235 = Index Array(array=w348, index=0) -> (element=w346:i32)
                n236 = for {
                  N: w346 -> [_]
                  tunnel: w345 -> [w356]
                  i -> [w354]
                  n237 = for {
                    N: 3 -> [_]
                    tunnel: w356 -> [w375]
                    tunnel: w354 -> [w369]
                    shift-right: [w372] -> w353
                    shift-left: "" -> [w374]
                    i -> [w368]
                    n238 = Index Array(array=w375, index (row)=w369, index (col)=w368) -> (element=w371:u16)
                    n239 = Quotient & Remainder(x=w371, y=10) -> (x-y*floor(x/y)=w366:i32)  [unwired: 1 out]
                    n240 = Increment(x=w366) -> (x+1=w367:i32)
                    n241 = Number To Decimal String(number=w367) -> (decimal integer string=w373:string)  [unwired: 1 in]
                    n242 = Concatenate Strings(w374, w373) -> (w372:string)
                  }
                  n243 = case shown="2" w354 {
                    tunnel: w353 -> [_ w358 w361 w364]
                    frame Default {
                    }
                    frame 0 {
                      n244 = property on="Chi 1" class="Bool (strict)"("Visible"=TRUE, "BoolText.Text"=w358, "BoolText.FontSize"=25) -> ()  [unwired: 2 in, 2 out]
                    }
                    frame 1 {
                      n245 = property on="Chi 2" class="Bool (strict)"("Visible"=TRUE, "BoolText.Text"=w361, "BoolText.FontSize"=25) -> ()  [unwired: 2 in, 2 out]
                    }
                    frame 2 {
                      n246 = property on="Chi 3" class="Bool (strict)"("Visible"=TRUE, "BoolText.Text"=w364, "BoolText.FontSize"=25) -> ()  [unwired: 2 in, 2 out]
                    }
                  }
                }
              }
            }
            n247 = Compound Arithmetic op=OR(w325, w324, w323, w322) -> (w321:bool)
            n248 = property on="Cancel" class="Bool (strict)"("Visible"=w321) -> ()  [unwired: 2 in, 2 out]
            n249 = case shown="False" w338 {
              tunnel: [4 w379] -> w337
              tunnel: w334 -> [w378 w380]
              tunnel: [T3."Interrupt0" T3."Draw"] -> w336
              tunnel: [w378 4] -> w335
              frame False {
              }
              frame True {
                n250 = call "GetNextPlayer.vi"("PlayerIndex"=w380) -> ("NewPlayerIndex"=w379:u16)  [unwired: 10 in]
              }
            }
          }
          frame "Interrupt0" {
            n251 = local read "Game"() -> (w387:T2)
            n252 = Unbundle By Name(w387) -> ("WhoHu"=w383:u16)
            n253 = Equal?(x=w383, y=4) -> (x = y?=w389:bool)
            n254 = case shown="False" w389 {
              tunnel: [T3."Hu?" T3."Interrupt1"] -> w385
              tunnel: [w390 4] -> w384
              tunnel: w383 -> [w390 _]
              frame False {
              }
              frame True {
              }
            }
          }
          frame "Interrupt1" {
            n255 = local read "Game"() -> (w400:T2)
            n256 = Unbundle By Name(w400) -> ("WhoKung"=w394:u16)
            n257 = Equal?(x=w394, y=4) -> (x = y?=w398:bool)
            n258 = case shown="False" w398 {
              tunnel: [w401 4] -> w397
              tunnel: [T3."Kung?" T3."Interrupt2"] -> w396
              tunnel: w394 -> [w401 _]
              frame False {
              }
              frame True {
              }
            }
          }
          frame "Interrupt2" {
            n259 = local read "Game"() -> (w411:T2)
            n260 = Unbundle By Name(w411) -> ("WhoPong"=w405:u16)
            n261 = Equal?(x=w405, y=4) -> (x = y?=w408:bool)
            n262 = case shown="True" w408 {
              tunnel: [T3."Pong?" T3."Interrupt3"] -> w407
              tunnel: [w412 4] -> w406
              tunnel: w405 -> [w412 _]
              frame False {
              }
              frame True {
              }
            }
          }
          frame "Interrupt3" {
            n263 = local read "Game"() -> (w423:T2)
            n264 = Unbundle By Name(w423) -> ("WhoChi"=w416:u16)
            n265 = Equal?(x=w416, y=4) -> (x = y?=w421:bool)
            n266 = case shown="False" w421 {
              tunnel: [w426 4] -> w420
              tunnel: [T3."Chi?" T3."Draw"] -> w419
              tunnel: w418 -> [w426 w427]
              tunnel: [w424 w428] -> w417
              tunnel: w416 -> [w424 _]
              frame False {
              }
              frame True {
                n267 = call "GetNextPlayer.vi"("PlayerIndex"=w427) -> ("NewPlayerIndex"=w428:u16)  [unwired: 10 in]
              }
            }
          }
          frame "Chi?" {
            n268 = local read "Players"() -> (w438:T1[])
            n269 = Index Array(array=w438, index=w431) -> (element=w437:T1)
            n270 = Unbundle By Name(w437) -> ("SelectedChi"=w435:i16)
            n271 = case shown="-1" w435 {
              selector: w435 -> [_ _ w447]
              tunnel: [T3."Chi?" T3."Draw" T3."Wait"] -> w433
              tunnel: [w439 w442 w446] -> w436
              tunnel: w431 -> [w439 w442 w446]
              tunnel: w434 -> [w440 _ w460]
              tunnel: [w440 4 4] -> w432
              frame -2, Default {
              }
              frame -1 {
              }
              frame 0..2 {
                w449 = FALSE
                n272 = local read "Players"() -> (w451:T1[])
                n273 = local write "Chi 1"(w449) -> ()
                n274 = local write "Chi 2"(w449) -> ()
                n275 = local write "Chi 3"(w449) -> ()
                n276 = Index Array(array=w451, index=w460) -> (element=w450:T1)
                n277 = local read "Players"() -> (w453:T1[])
                n278 = Index Array(array=w453, index=w446) -> (element=w454:T1)
                n279 = call "DeleteTileFromRiver.vi"("Player"=w450) -> ("DeletedTile"=w455:u16, "NewPlayer"=w452:T1)  [unwired: 9 in]
                n280 = Replace Array Subset(array=w451, new element=w452, index=w460) -> (w445:T1[])
                n281 = for {
                  N: 3 -> [_]
                  shift-right: [w463] -> w456
                  shift-left: w454 -> [w464]
                  tunnel: w455 -> [w462]
                  tunnel: w447 -> [w461]
                  i -> [w465]
                  n282 = case shown="0, 2" w465 {
                    selector: w465 -> [_ w474]
                    tunnel: w464 -> [w471 w476]
                    tunnel: [w472 w475] -> w463
                    tunnel: w462 -> [w470 _]
                    tunnel: w461 -> [_ w473]
                    frame 1, Default {
                      n283 = Unbundle By Name(w471) -> ("Door"=w469:u16[], "DoorCount"=w466:u16)
                      n284 = Replace Array Subset(array=w469, new element=w470, index=w466) -> (w468:u16[])
                      n285 = Increment(x=w466) -> (x+1=w467:u16)
                      n286 = Bundle By Name(cluster=w471, "Door"=w468, "DoorCount"=w467) -> (w472:T1)
                    }
                    frame 0, 2 {
                      n287 = Unbundle By Name(w476) -> ("ChiChoice"=w478:u16[][])
                      n288 = Index Array(array=w478, index (row)=w473, index (col)=w474) -> (element=w477:u16)
                      n289 = call "DeleteFromHandAndAddToDoor.vi"("Tile"=w477, "Player"=w476) -> ("NewPlayer"=w475:T1)  [unwired: 9 in]
                    }
                  }
                }
                n290 = Replace Array Subset(array=w445, new element=w456, index=w446) -> (w457:T1[])
                n291 = local write "Players"(w457) -> ()
              }
            }
          }
          frame "Pong?" {
            n292 = local read "Players"() -> (w486:T1[])
            n293 = Index Array(array=w486, index=w480) -> (element=w485:T1)
            n294 = Unbundle By Name(w485) -> ("SelectedPong"=w479:i16)
            n295 = case shown="1" w479 {
              tunnel: [T3."Pong?" T3."Interrupt3" T3."Wait"] -> w484
              tunnel: [w489 w492 4] -> w483
              tunnel: [w487 w491 w503] -> w482
              tunnel: w480 -> [w487 w491 w503]
              tunnel: w481 -> [w489 w492 w509]
              frame -2, Default {
              }
              frame -1 {
              }
              frame 1 {
                n296 = local read "Players"() -> (w508:T1[])
                n297 = Index Array(array=w508, index=w509) -> (element=w511:T1)
                n298 = Index Array(array=w508, index=w503) -> (element=w506:T1)
                n299 = call "DeleteTileFromRiver.vi"("Player"=w511) -> ("DeletedTile"=w494:u16, "NewPlayer"=w510:T1)  [unwired: 9 in]
                n300 = Replace Array Subset(array=w508, new element=w510, index=w509) -> (w493:T1[])
                n301 = for {
                  N: 2 -> [_]
                  tunnel: w494 -> [w515]
                  shift-right: [w514] -> w505
                  shift-left: w506 -> [w516]
                  n302 = call "DeleteFromHandAndAddToDoor.vi"("Tile"=w515, "Player"=w516) -> ("NewPlayer"=w514:T1)  [unwired: 9 in]
                }
                n303 = Unbundle By Name(w505) -> ("Door"=w501:u16[], "DoorCount"=w498:u16, "Ponged"=w495:u16[])
                n304 = Replace Array Subset(array=w501, new element=w494, index=w498) -> (w499:u16[])
                n305 = Array Size(array=w495) -> (size(s)=w496:i32)
                n306 = Insert Into Array(array=w495, index=w496, new element=w494) -> (w497:u16[])
                n307 = Increment(x=w498) -> (x+1=w500:u16)
                n308 = Bundle By Name(cluster=w505, "Door"=w499, "DoorCount"=w500, "Ponged"=w497) -> (w504:T1)
                n309 = Replace Array Subset(array=w493, new element=w504, index=w503) -> (w502:T1[])
                n310 = local write "Players"(w502) -> ()
              }
            }
          }
          frame "Kung?" {
            n311 = local read "Players"() -> (w524:T1[])
            n312 = Index Array(array=w524, index=w518) -> (element=w523:T1)
            n313 = Unbundle By Name(w523) -> ("SelectedKung"=w517:i16)
            n314 = case shown="1" w517 {
              tunnel: [T3."Kung?" T3."Interrupt2" T3."Draw"] -> w522
              tunnel: [w526 w530 4] -> w521
              tunnel: [w525 w529 w538] -> w520
              tunnel: w518 -> [w525 w529 w538]
              tunnel: w519 -> [w526 w530 w544]
              frame -2, Default {
              }
              frame -1 {
              }
              frame 1 {
                n315 = local read "Players"() -> (w543:T1[])
                n316 = Index Array(array=w543, index=w544) -> (element=w546:T1)
                n317 = Index Array(array=w543, index=w538) -> (element=w541:T1)
                n318 = call "DeleteTileFromRiver.vi"("Player"=w546) -> ("DeletedTile"=w534:u16, "NewPlayer"=w545:T1)  [unwired: 9 in]
                n319 = Replace Array Subset(array=w543, new element=w545, index=w544) -> (w531:T1[])
                n320 = for {
                  N: 3 -> [_]
                  shift-right: [w549] -> w540
                  shift-left: w541 -> [w550]
                  tunnel: w534 -> [w551]
                  n321 = call "DeleteFromHandAndAddToDoor.vi"("Tile"=w551, "Player"=w550) -> ("NewPlayer"=w549:T1)  [unwired: 9 in]
                }
                n322 = Unbundle By Name(w540) -> ("Door"=w536:u16[], "DoorCount"=w532:u16)
                n323 = Replace Array Subset(array=w536, new element=w534, index=w532) -> (w535:u16[])
                n324 = Increment(x=w532) -> (x+1=w533:u16)
                n325 = Bundle By Name(cluster=w540, "Door"=w535, "DoorCount"=w533) -> (w539:T1)
                n326 = Replace Array Subset(array=w531, new element=w539, index=w538) -> (w537:T1[])
                n327 = local write "Players"(w537) -> ()
              }
            }
          }
          frame "Hu?" {
            n328 = local read "Players"() -> (w559:T1[])
            n329 = Index Array(array=w559, index=w552) -> (element=w558:T1)
            n330 = Unbundle By Name(w558) -> ("SelectedHu"=w557:i16)
            n331 = case shown="-1" w557 {
              tunnel: [T3."Hu?" T3."Interrupt1" T3."Game End"] -> w556
              tunnel: [w562 w565 w566] -> w555
              tunnel: [w560 w564 w567] -> w554
              tunnel: w552 -> [w560 w564 w567]
              tunnel: w553 -> [w562 w565 w566]
              frame -2, Default {
              }
              frame -1 {
              }
              frame 1 {
              }
            }
          }
          frame Default {
          }
        }
      }
      frame #1 {
        n332 = case shown="\"Chi?\"" w574 {
          tunnel: w572 -> [_ w577 _ _ _ _]
          frame Default {
          }
          frame "Wait" {
            n333 = Equal To 0?(x=w577) -> (x = 0?=w578:bool)
            n334 = local read "Players"() -> (w584:T1[])
            n335 = Index Array(array=w584, index=w577) -> (element=w579:T1)
            n336 = case shown="True" w578 {
              tunnel: w579 -> [w598 w632]
              tunnel: [w595 w626] -> w582
              tunnel: w577 -> [_ w615]
              tunnel: [w591 w614] -> w576
              tunnel: [w594 w613] -> w575
              frame False {
                n337 = local read "Game"() -> (w593:T2)
                n338 = Unbundle By Name(w598) -> ("Hand"=w597:u16[], "HandCount"=w596:u16, "KungChoice"=w592:u16)
                n339 = Unbundle By Name(w593) -> ("WhoKung"=w589:u16, "WhoHu"=w585:u16)
                n340 = Not Equal?(x=w585, y=4) -> (x != y?=w587:bool)
                n341 = Not Equal?(x=w589, y=4) -> (x != y?=w590:bool)
                n342 = case shown="True" w587 {
                  tunnel: [-1 w602] -> w594
                  frame False {
                  }
                  frame True {
                    n343 = call "HuStrategy.vi"() -> ("Hu?"=w603:bool)  [unwired: 11 in]
                    n344 = Select(t=1, s=w603, f=-1) -> (s? t:f=w602:i32)
                  }
                }
                n345 = case shown="True" w590 {
                  tunnel: w592 -> [_ w606]
                  tunnel: [-1 w605] -> w591
                  frame False {
                  }
                  frame True {
                    n346 = call "KungStrategy.vi"("TargetTile"=w606) -> ("Kung?"=w609:bool)  [unwired: 10 in]
                    n347 = Select(t=1, s=w609, f=-1) -> (s? t:f=w605:i32)
                  }
                }
                n348 = call "ThrowTile.vi"("HandSize"=w596, "Hand"=w597) -> ("Which"=w595:u16)
              }
              frame True {
                n349 = Unbundle By Name(w632) -> ("HandCount"=w624:u16, "SelectedTile"=w625:i16, "Kung"=w616:bool, "Hu"=w611:bool, "Cancel"=w610:bool)
                n350 = local read "Game"() -> (w622:T2)
                n351 = Unbundle By Name(w622) -> ("WhoKung"=w621:u16, "WhoHu"=w612:u16)
                n352 = local read "Buttons"() -> (w634:bool[])
                n353 = Not Equal?(x=w625, y=-1) -> (x != y?=w629:bool)
                n354 = Not Equal?(x=w612, y=u16 4) -> (x != y?=w617:bool)
                n355 = Not Equal?(x=w621, y=u16 4) -> (x != y?=w619:bool)
                n356 = Search 1D Array(1D array=w634, element=TRUE) -> (index of element=w623:i32)  [unwired: 1 in]
                n357 = case shown="True" w617 {
                  tunnel: [-1 w636] -> w613
                  tunnel: w611 -> [_ w641]
                  tunnel: w610 -> [_ w638]
                  frame False {
                  }
                  frame True {
                    n358 = Select(t=1, s=w641, f=-2) -> (s? t:f=w639:i32)
                    n359 = Select(t=-1, s=w638, f=w639) -> (s? t:f=w636:i32)
                  }
                }
                n360 = case shown="True" w619 {
                  tunnel: w616 -> [_ w650]
                  tunnel: w615 -> [_ _]
                  tunnel: [-1 w647] -> w614
                  tunnel: w610 -> [_ w646]
                  frame False {
                  }
                  frame True {
                    n361 = Select(t=1, s=w650, f=-2) -> (s? t:f=w645:i32)
                    n362 = Select(t=-1, s=w646, f=w645) -> (s? t:f=w647:i32)
                  }
                }
                n363 = Less?(x=w623, y=w624) -> (x < y?=w631:bool)
                n364 = Select(t=w623, s=w631, f=-1) -> (s? t:f=w627:i32)
                n365 = Select(t=w625, s=w629, f=w627) -> (s? t:f=w626:i32)
              }
            }
            n366 = local read "Players"() -> (w583:T1[])
            n367 = Bundle By Name(cluster=w579, "SelectedTile"=w582, "SelectedKung"=w576, "SelectedHu"=w575) -> (w581:T1)
            n368 = Replace Array Subset(array=w583, new element=w581, index=w577) -> (w580:T1[])
            n369 = local write "Players"(w580) -> ()
          }
          frame "Chi?" {
            n370 = local read "Game"() -> (w652:T2)
            n371 = local read "Players"() -> (w657:T1[])
            n372 = Unbundle By Name(w652) -> ("WhoChi"=w651:u16)
            n373 = Index Array(array=w657, index=w651) -> (element=w654:T1)
            n374 = Equal To 0?(x=w651) -> (x = 0?=w658:bool)
            n375 = case shown="False" w658 {
              tunnel: w654 -> [w664 w672]
              tunnel: [w660 w669] -> w653
              frame False {
                n376 = Unbundle By Name(w664) -> ("Hand"=w663:u16[], "ChiChoice"=w662:u16[][])
                n377 = call "ChiStrategy.vi"("ChiChoice"=w662, "Hand"=w663) -> ("Result"=w660:i16)  [unwired: 9 in]
                n378 = Not Equal?(x=w660, y=-1) -> (x != y?=w661:bool)
                n379 = case shown="True" w661 {
                  frame False {
                  }
                  frame True {
                    n380 = Current VI's Path() -> (path=w666:path)
                    n381 = Strip Path(path=w666) -> (stripped path=w667:path)  [unwired: 1 out]
                    n382 = Build Path(base path=w667, name or relative path=path "Sounds/chi.wav") -> (appended path=w668:path)
                    n383 = call <vilib>:"Play Sound File.vi"("path"=w668) -> ()  [unwired: 9 in, 2 out]
                  }
                }
              }
              frame True {
                n384 = Unbundle By Name(w672) -> ("Chi"=w671:bool, "Cancel"=w670:bool)
                n385 = case shown="True" w671 {
                  tunnel: w670 -> [w674 _]
                  tunnel: [w673 w679] -> w669
                  frame False {
                    n386 = case shown="False" w674 {
                      tunnel: [-2 -1] -> w673
                      frame False {
                      }
                      frame True {
                      }
                    }
                  }
                  frame True {
                    n387 = local read "Chi 1"() -> (w686:bool)
                    n388 = local read "Chi 3"() -> (w684:bool)
                    n389 = local read "Chi 2"() -> (w685:bool)
                    n390 = Build Array(w686, w685, w684) -> (w683:bool[])
                    n391 = Search 1D Array(1D array=w683, element=TRUE) -> (index of element=w678:i32)  [unwired: 1 in]
                    n392 = Equal?(x=w678, y=-1) -> (x = y?=w677:bool)
                    n393 = case shown="False" w677 {
                      frame False {
                        n394 = Current VI's Path() -> (path=w690:path)
                        n395 = Strip Path(path=w690) -> (stripped path=w689:path)  [unwired: 1 out]
                        n396 = Build Path(base path=w689, name or relative path=path "Sounds/chi.wav") -> (appended path=w687:path)
                        n397 = call <vilib>:"Play Sound File.vi"("path"=w687) -> ()  [unwired: 9 in, 2 out]
                      }
                      frame True {
                      }
                    }
                    n398 = Select(t=-2, s=w677, f=w678) -> (s? t:f=w679:i32)
                  }
                }
              }
            }
            n399 = Bundle By Name(cluster=w654, "SelectedChi"=w653) -> (w656:T1)
            n400 = Replace Array Subset(array=w657, new element=w656, index=w651) -> (w655:T1[])
            n401 = local write "Players"(w655) -> ()
          }
          frame "Pong?" {
            n402 = local read "Game"() -> (w692:T2)
            n403 = local read "Players"() -> (w697:T1[])
            n404 = Unbundle By Name(w692) -> ("WhoPong"=w691:u16)
            n405 = Equal To 0?(x=w691) -> (x = 0?=w695:bool)
            n406 = Index Array(array=w697, index=w691) -> (element=w694:T1)
            n407 = case shown="False" w695 {
              tunnel: w694 -> [w705 w713]
              tunnel: [w702 w710] -> w693
              frame False {
                n408 = Unbundle By Name(w705) -> ("Hand"=w704:u16[], "PongChoice"=w703:u16)
                n409 = call "PongStrategy.vi"("TargetTile"=w703, "Hand"=w704) -> ("Pong?"=w699:bool)  [unwired: 9 in]
                n410 = case shown="True" w699 {
                  frame False {
                  }
                  frame True {
                    n411 = Current VI's Path() -> (path=w709:path)
                    n412 = Strip Path(path=w709) -> (stripped path=w708:path)  [unwired: 1 out]
                    n413 = Build Path(base path=w708, name or relative path=path "Sounds/pon.wav") -> (appended path=w707:path)
                    n414 = call <vilib>:"Play Sound File.vi"("path"=w707) -> ()  [unwired: 9 in, 2 out]
                  }
                }
                n415 = Select(t=1, s=w699, f=-1) -> (s? t:f=w702:i32)
              }
              frame True {
                n416 = Unbundle By Name(w713) -> ("Pong"=w712:bool, "Cancel"=w711:bool)
                n417 = case shown="True" w712 {
                  tunnel: w711 -> [w715 _]
                  tunnel: [w714 1] -> w710
                  frame False {
                    n418 = case shown="True" w715 {
                      tunnel: [-2 -1] -> w714
                      frame False {
                      }
                      frame True {
                      }
                    }
                  }
                  frame True {
                    n419 = Current VI's Path() -> (path=w722:path)
                    n420 = Strip Path(path=w722) -> (stripped path=w721:path)  [unwired: 1 out]
                    n421 = Build Path(base path=w721, name or relative path=path "Sounds/pon.wav") -> (appended path=w720:path)
                    n422 = call <vilib>:"Play Sound File.vi"("path"=w720) -> ()  [unwired: 9 in, 2 out]
                  }
                }
              }
            }
            n423 = Bundle By Name(cluster=w694, "SelectedPong"=w693) -> (w698:T1)
            n424 = Replace Array Subset(array=w697, new element=w698, index=w691) -> (w696:T1[])
            n425 = local write "Players"(w696) -> ()
          }
          frame "Kung?" {
            n426 = local read "Game"() -> (w724:T2)
            n427 = Unbundle By Name(w724) -> ("WhoKung"=w723:u16)
            n428 = Equal To 0?(x=w723) -> (x = 0?=w727:bool)
            n429 = local read "Players"() -> (w730:T1[])
            n430 = Index Array(array=w730, index=w723) -> (element=w726:T1)
            n431 = case shown="False" w727 {
              tunnel: w726 -> [w734 w745]
              tunnel: [w737 w742] -> w725
              frame False {
                n432 = Unbundle By Name(w734) -> ("Hand"=w733:u16[], "KungChoice"=w732:u16)
                n433 = call "KungStrategy.vi"("TargetTile"=w732, "Hand"=w733) -> ("Kung?"=w731:bool)  [unwired: 9 in]
                n434 = case shown="True" w731 {
                  frame False {
                  }
                  frame True {
                    n435 = Current VI's Path() -> (path=w741:path)
                    n436 = Strip Path(path=w741) -> (stripped path=w740:path)  [unwired: 1 out]
                    n437 = Build Path(base path=w740, name or relative path=path "Sounds/kan.wav") -> (appended path=w739:path)
                    n438 = call <vilib>:"Play Sound File.vi"("path"=w739) -> ()  [unwired: 9 in, 2 out]
                  }
                }
                n439 = Select(t=1, s=w731, f=-1) -> (s? t:f=w737:i32)
              }
              frame True {
                n440 = Unbundle By Name(w745) -> ("Kung"=w744:bool, "Cancel"=w743:bool)
                n441 = case shown="True" w744 {
                  tunnel: w743 -> [w747 _]
                  tunnel: [w746 1] -> w742
                  frame False {
                    n442 = case shown="False" w747 {
                      tunnel: [-2 -1] -> w746
                      frame False {
                      }
                      frame True {
                      }
                    }
                  }
                  frame True {
                    n443 = Current VI's Path() -> (path=w753:path)
                    n444 = Strip Path(path=w753) -> (stripped path=w752:path)  [unwired: 1 out]
                    n445 = Build Path(base path=w752, name or relative path=path "Sounds/kan.wav") -> (appended path=w751:path)
                    n446 = call <vilib>:"Play Sound File.vi"("path"=w751) -> ()  [unwired: 9 in, 2 out]
                  }
                }
              }
            }
            n447 = Bundle By Name(cluster=w726, "SelectedKung"=w725) -> (w728:T1)
            n448 = Replace Array Subset(array=w730, new element=w728, index=w723) -> (w729:T1[])
            n449 = local write "Players"(w729) -> ()
          }
          frame "Hu?" {
            n450 = local read "Game"() -> (w756:T2)
            n451 = local read "Players"() -> (w761:T1[])
            n452 = Unbundle By Name(w756) -> ("WhoHu"=w755:u16)
            n453 = Equal To 0?(x=w755) -> (x = 0?=w759:bool)
            n454 = Index Array(array=w761, index=w755) -> (element=w758:T1)
            n455 = case shown="False" w759 {
              tunnel: w758 -> [_ w770]
              tunnel: [w763 w767] -> w757
              frame False {
                n456 = call "HuStrategy.vi"() -> ("Hu?"=w766:bool)  [unwired: 11 in]
                n457 = Select(t=1, s=w766, f=-1) -> (s? t:f=w763:i32)
              }
              frame True {
                n458 = Unbundle By Name(w770) -> ("Hu"=w769:bool, "Cancel"=w768:bool)
                n459 = case shown="False" w769 {
                  selector: w769 -> [_ w778]
                  tunnel: w768 -> [w772 _]
                  tunnel: [w771 w777] -> w767
                  frame False {
                    n460 = case shown="False" w772 {
                      tunnel: [-2 -1] -> w771
                      frame False {
                      }
                      frame True {
                      }
                    }
                  }
                  frame True {
                    n461 = Select(t=1, s=w778, f=-2) -> (s? t:f=w777:i32)
                  }
                }
              }
            }
            n462 = Bundle By Name(cluster=w758, "SelectedHu"=w757) -> (w760:T1)
            n463 = Replace Array Subset(array=w761, new element=w760, index=w755) -> (w762:T1[])
            n464 = local write "Players"(w762) -> ()
          }
        }
      }
      frame #2 {
        n465 = case shown="Default" w779 {
          frame "Game End" {
          }
          frame Default {
            n466 = local read "Players"() -> (w803:T1[])
            n467 = Index Array(array=w803, index=1) -> (element=w816:T1)
            n468 = Index Array(array=w803, index=2) -> (element=w827:T1)
            n469 = Index Array(array=w803, index=0) -> (element=w832:T1)
            n470 = Index Array(array=w803, index=3) -> (element=w813:T1)
            n471 = Unbundle By Name(w816) -> ("HandCount"=w783:u16, "River"=w811:u16[][], "Door"=w819:u16[])
            n472 = Unbundle By Name(w827) -> ("HandCount"=w790:u16, "River"=w806:u16[][], "Door"=w824:u16[])
            n473 = Unbundle By Name(w813) -> ("HandCount"=w802:u16, "River"=w810:u16[][], "Door"=w812:u16[])
            n474 = Unbundle By Name(w832) -> ("Hand"=w830:u16[], "River"=w831:u16[][], "Door"=w833:u16[])
            n475 = Initialize Array(38, w790) -> (w795:i32[])
            n476 = Initialize Array(38, w783) -> (w788:i32[])
            n477 = Initialize Array(37, 17) -> (w794:i32[])
            n478 = local write "Hand1"(w830) -> ()
            n479 = Array Subset(array=w819, length=19) -> (w820:u16[])  [unwired: 1 in]
            n480 = local write "River1"(w831) -> ()
            n481 = local write "Door1"(w833) -> ()
            n482 = Array Subset(array=w824, length=19) -> (w823:u16[])  [unwired: 1 in]
            n483 = Initialize Array(37, 17) -> (w787:i32[])
            n484 = Initialize Array(38, w802) -> (w796:i32[])
            n485 = Replace Array Subset(array=w794, new element=w795) -> (w789:i32[])  [unwired: 1 in]
            n486 = Reverse 1D Array(array=w820) -> (reversed array=w821:u16[])
            n487 = Replace Array Subset(array=w787, new element=w788) -> (w782:i32[])  [unwired: 1 in]
            n488 = Reverse 1D Array(array=w823) -> (reversed array=w822:u16[])
            n489 = Transpose 2D Array(2D array=w811) -> (transposed array=w809:u16[][])
            n490 = Initialize Array(37, 17) -> (w798:i32[])
            n491 = Reverse 1D Array(array=w789) -> (reversed array=w826:i32[])
            n492 = local write "Door4"(w812) -> ()
            n493 = Reverse 1D Array(array=w782) -> (reversed array=w817:i32[])
            n494 = Transpose 2D Array(2D array=w810) -> (transposed array=w804:u16[][])
            n495 = Replace Array Subset(array=w798, new element=w796) -> (w797:i32[])  [unwired: 1 in]
            n496 = local write "Hand3"(w826) -> ()
            n497 = local write "Door2"(w821) -> ()
            n498 = local write "Door3"(w822) -> ()
            n499 = local write "Hand2"(w817) -> ()
            n500 = local write "Hand4"(w797) -> ()
            n501 = for {
              N: 3 -> [_]
              tunnel: w809 -> [w859]
              i -> [w858]
              n502 = for {
                N: 12 -> [_]
                tunnel: w859 -> [w868]
                tunnel: w858 -> [w865]
                i -> [w862]
                n503 = Index Array(array=w868, index (row)=w862, index (col)=w865) -> (element=w864:u16)
                n504 = local read "River2"() -> (w866:u16[][])
                n505 = Subtract(x=11 ("y"), y=w862) -> (x-y=w863:i32)
                n506 = Replace Array Subset(array=w866, new element=w864, index (row)=w863, index (col)=w865) -> (w867:u16[][])
                n507 = local write "River2"(w867) -> ()
              }
            }
            n508 = for {
              N: 3 -> [_]
              tunnel: w806 -> [w846]
              i -> [w845]
              n509 = for {
                N: 12 -> [_]
                tunnel: w846 -> [w857]
                tunnel: w845 -> [w850]
                i -> [w851]
                n510 = Index Array(array=w857, index (row)=w850, index (col)=w851) -> (element=w852:u16)
                n511 = local read "River 3"() -> (w855:u16[][])
                n512 = Subtract(x=2, y=w850) -> (x-y=w848:i32)
                n513 = Subtract(x=11 ("y"), y=w851) -> (x-y=w849:i32)
                n514 = Replace Array Subset(array=w855, new element=w852, index (row)=w848, index (col)=w849) -> (w856:u16[][])
                n515 = local write "River 3"(w856) -> ()
              }
            }
            n516 = for {
              N: 3 -> [_]
              tunnel: w804 -> [w835]
              i -> [w834]
              n517 = for {
                N: 12 -> [_]
                tunnel: w835 -> [w844]
                tunnel: w834 -> [w839]
                i -> [w837]
                n518 = Index Array(array=w844, index (row)=w837, index (col)=w839) -> (element=w841:u16)
                n519 = local read "River4"() -> (w842:u16[][])
                n520 = Subtract(x=2, y=w839) -> (x-y=w840:i32)
                n521 = Replace Array Subset(array=w842, new element=w841, index (row)=w837, index (col)=w840) -> (w843:u16[][])
                n522 = local write "River4"(w843) -> ()
              }
            }
          }
        }
      }
    }
    n523 = Index Array(array=w18, index=w10) -> (element=w19:T1)
    n524 = local read "Cancel"() -> (w12:bool)
    n525 = local read "Pong"() -> (w13:bool)
    n526 = local read "Kung"() -> (w14:bool)
    n527 = local read "Chi"() -> (w16:bool)
    n528 = local read "Hu"() -> (w15:bool)
    n529 = Bundle By Name(cluster=w19, "Chi"=w16, "Pong"=w13, "Kung"=w14, "Hu"=w15, "Cancel"=w12) -> (w17:T1)
    n530 = Replace Array Subset(array=w18, new element=w17, index=w10) -> (w20:T1[])
    n531 = local write "Players"(w20) -> ()
  }
